vi "varXNode_Mutate_8_5_0_0.vi"(8 "error in (no error)":errorcluster, 9 "Replies in":string[](array[string]), 10 "Version":T1, 11 "Old State":variant) -> (0 "error out":errorcluster, 1 "Replies out":string[](array[string]), 2 "Version Out":T1, 3 "New State":variant)   [LabVIEW 2020, in "varXNode.xnode"]
uses:
  <vilib>/variable/varXNode.llb/varXNode.xnode
  <vilib>/XNodeSupport/XNodeVersion.ctl
  <vilib>/XNodeSupport/XNodeUShort.ctl
  <vilib>/variable/varXNode.llb/varXNode.ctl
  <vilib>/variable/Type Descriptor.ctl
  <vilib>/variable/varXNode.llb/varXNode_old_8_1_0_1.ctl
  <vilib>/XNodeSupport/NI_XNodeSupport.lvlib
  <vilib>/variable/NI_Variable.lvlib
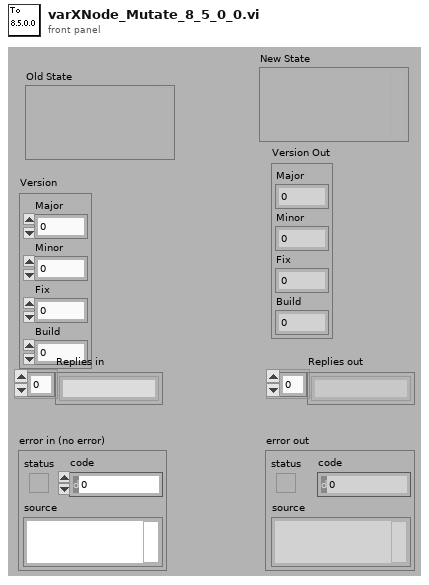
[diagram p1: front panel]
types:
  T1 = typedef "NI_XNodeSupport.lvlib/XNodeVersion.ctl" = cluster{"Major":T2, "Minor":T2, "Fix":T2, "Build":T2}
  T2 = typedef "NI_XNodeSupport.lvlib/XNodeUShort.ctl" = u16
  T3 = typedef "varXNode.xnode/varXNode_old_8_1_0_1.ctl" = cluster{"Write":bool, "ShowTimestamp":bool, "CachedName":string, "CachedTypeDesc":T4, "CachedFeaturePacks":string[], "Custom Rule":string, "ProjectPath":string, "Bad Code":bool, "ContextName":string, "Allow Timestamp":bool, "Generate Code?":bool}
  T4 = typedef "NI_Variable.lvlib/Type Descriptor.ctl" = cluster{"Variant":variant}
  T5 = typedef "varXNode.xnode/varXNode.ctl" = cluster{"Write":bool, "ShowTimestamp":bool, "CachedName":string, "CachedTypeDesc":T4, "CachedFeaturePacks":string[], "Custom Rule":string, "ProjectPath":string, "Bad Code":bool, "ContextName":string, "Allow Timestamp":bool, "Generate Code?":bool, "targetRelative?":bool}
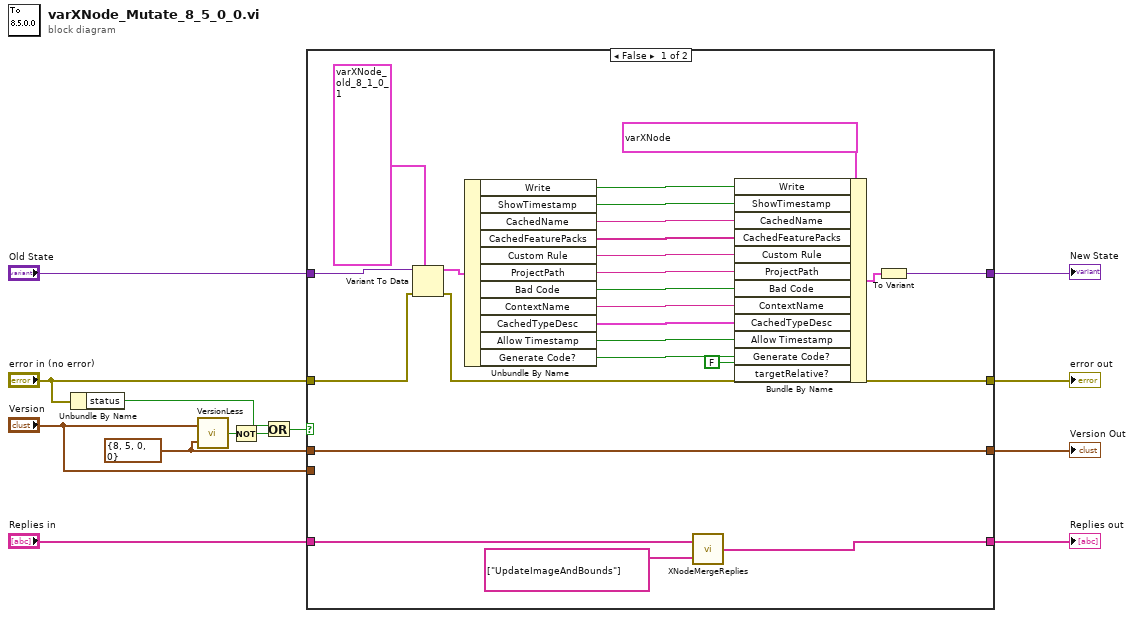
[diagram p0: block diagram]
diagram:
  w12 = T1 {"Major"=8, "Minor"=5, "Fix"=0, "Build"=0} ("y")
  n1 = Unbundle By Name("error in (no error)") -> ("status"=w4:bool)
  n2 = call <vilib>:"VersionLess.vi"("y"=w12, "x"="Version") -> ("x < y?"=w13:bool)
  n3 = Not(x=w13) -> (.not. x?=w3:bool)
  n4 = Or(x=w4, y=w3) -> (x .or. y?=w6:bool)
  n5 = case shown="False" w6 {
    tunnel: w12 -> [w37 _]
    tunnel: [w26 w41] -> w11
    tunnel: "Old State" -> [w36 w41]
    tunnel: [w37 w40] -> w9
    tunnel: "Version" -> [_ w40]
    tunnel: [w21 w39] -> w7
    tunnel: "error in (no error)" -> [w22 w39]
    tunnel: [w15 w38] -> w2
    tunnel: "Replies in" -> [w16 w38]
    frame False {
      n6 = Variant To Data(error in=w22, type=T3 {"Write"=FALSE, "ShowTimestamp"=FALSE, "CachedName"="", "CachedTypeDesc"={"Variant"=variant}, "CachedFeaturePacks"=[], "Custom Rule"="", "ProjectPath"="", "Bad Code"=FALSE, "ContextName"="", "Allow Timestamp"=FALSE, "Generate Code?"=FALSE} ("State"), Variant=w36) -> (data=w20:T3, error out=w21:errorcluster)
      n7 = Unbundle By Name(w20) -> ("Write"=w34:bool, "ShowTimestamp"=w33:bool, "CachedName"=w32:string, "CachedFeaturePacks"=w31:string[], "Custom Rule"=w30:string, "ProjectPath"=w29:string, "Bad Code"=w28:bool, "ContextName"=w27:string, "CachedTypeDesc"=w23:T4, "Allow Timestamp"=w19:bool, "Generate Code?"=w18:bool)
      n8 = call <vilib>:"XNodeMergeReplies.vi"("New Replies"=string[] ["UpdateImageAndBounds"], "Old Replies"=w16) -> ("Merged Replies"=w15:string[])
      n9 = Bundle By Name(cluster=T5 {"Write"=FALSE, "ShowTimestamp"=FALSE, "CachedName"="", "CachedTypeDesc"={"Variant"=variant}, "CachedFeaturePacks"=[], "Custom Rule"="", "ProjectPath"="", "Bad Code"=FALSE, "ContextName"="", "Allow Timestamp"=FALSE, "Generate Code?"=FALSE, "targetRelative?"=FALSE} ("State"), "Write"=w34, "ShowTimestamp"=w33, "CachedName"=w32, "CachedFeaturePacks"=w31, "Custom Rule"=w30, "ProjectPath"=w29, "Bad Code"=w28, "ContextName"=w27, "CachedTypeDesc"=w23, "Allow Timestamp"=w19, "Generate Code?"=w18, "targetRelative?"=FALSE ("Local Reference?")) -> (w25:T5)
      n10 = To Variant(anything=w25) -> (Variant=w26:variant)
    }
    frame True {
      # "Either there was an error in,\nor the version is not less than 1.0.0.6.\nPass input values out."
    }
  }
  "New State" <- w11
  "Version Out" <- w9
  "error out" <- w7
  "Replies out" <- w2
